vi "MPM_Set_Range_Each_Channel.vi"(6 "Range for each ch":i32, 8 "error in (no error)":errorcluster, 9 "Ch":i32, 10 "Slot":i32, 11 ".NET Reference in":refnum<k24>) -> (0 "error out":errorcluster, 3 "Reference out":refnum<k24>)   [LabVIEW 2017]
uses:
  C:/Users/Ssantec_Test/Documents/Instrument_DLL_Sample_Labview_20250826_Ver1.5.0_x64/DLL/InstrumentDLL.dll
  DLL/InstrumentDLL.dll
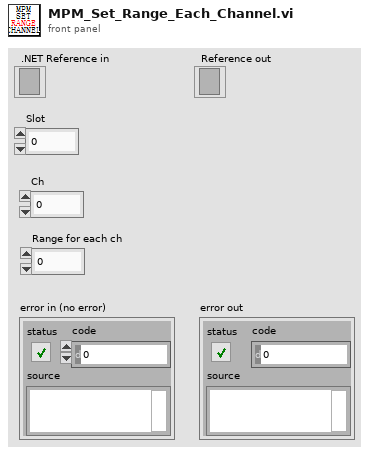
[diagram p1: front panel]
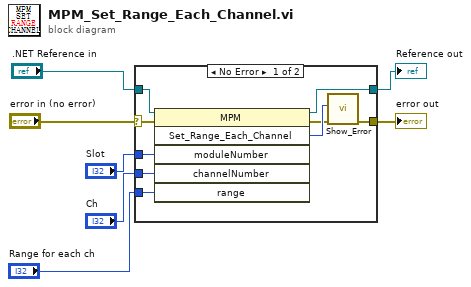
[diagram p0: block diagram]
diagram:
  n1 = case shown="No Error" "error in (no error)" {
    selector: "error in (no error)" -> [w8 w17]
    tunnel: "Range for each ch" -> [w16 _]
    tunnel: "Ch" -> [w15 _]
    tunnel: "Slot" -> [w14 _]
    tunnel: ".NET Reference in" -> [w13 w18]
    tunnel: [w12 w18] -> w3
    tunnel: [w9 w17] -> w2
    frame No Error {
      n2 = invoke on="调用节点" class="MPM" method="Set_Range_Each_Channel"(reference=w13, error in=w8, "moduleNumber"=w14, "channelNumber"=w15, "range"=w16) -> (reference out=w12:refnum<k24>, error out=w10:errorcluster, "Set_Range_Each_Channel"=w11:i32)  [unwired: 1 in, 3 out]
      n3 = call "Show_Error.vi"("error in (no error)"=w10, "Error"=w11) -> ("error out"=w9:errorcluster)  [unwired: 9 in]
    }
    frame Error {
    }
  }
  "Reference out" <- w3
  "error out" <- w2
